vi "Select Path.vi"(8 "error in":errorcluster) -> (0 "error out":errorcluster, 1 "Save?":bool, 2 "selected path":path, 3 "Path":string)   [LabVIEW 2014, in "Data Saving.lvlib" / "Data Saver.lvclass"]
uses:
  Data Saver.lvclass
  Data Logger/PathFinder Type def.ctl
  Data Logger/Data Logger.lvclass
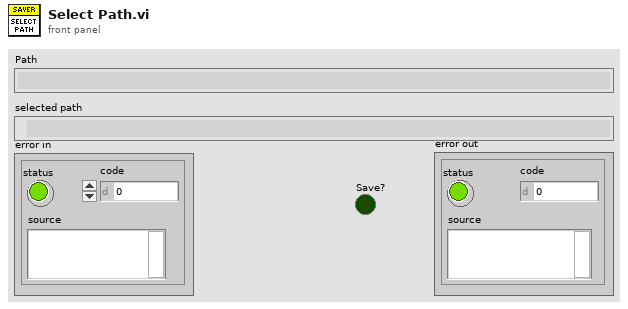
[diagram p1: front panel]
types:
  T1 = typedef "PathFinder Type def.ctl" = enum16{"Done", "Waiting"}
  T2 = cluster{"Project Number":string, "Manufacturer":string, "Model":string, "Serial":string, "Comment":string}
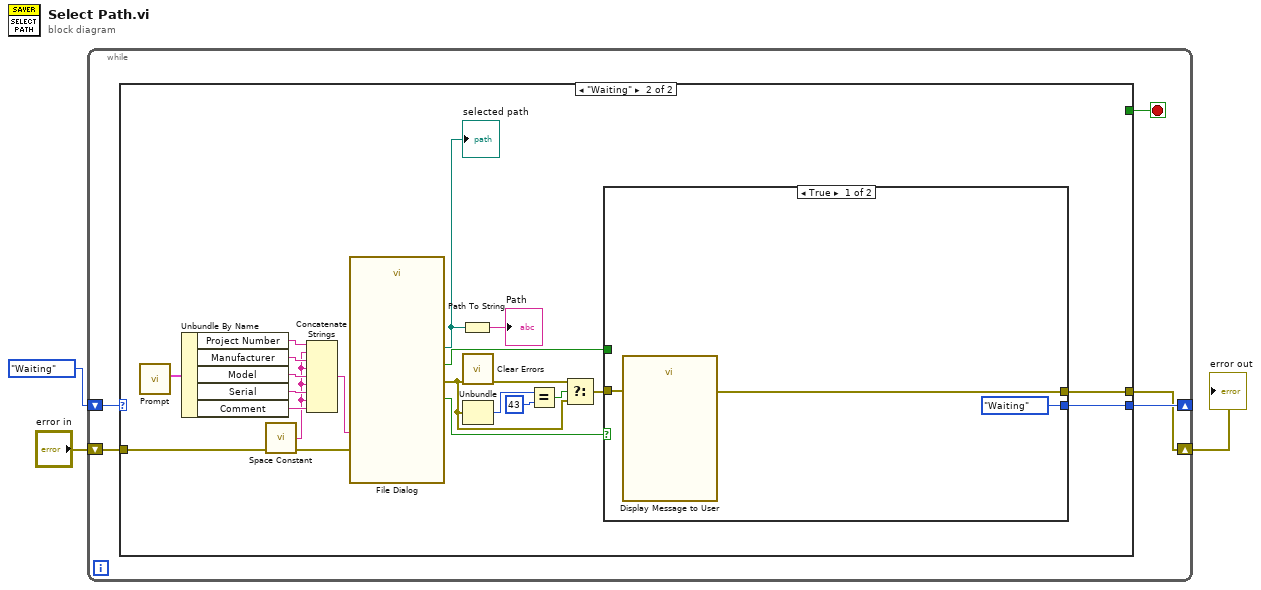
[diagram p0: block diagram]
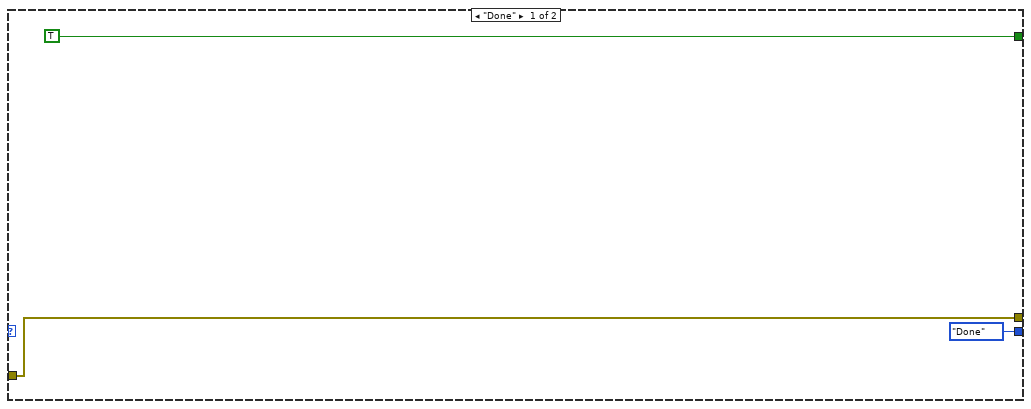
[diagram p2: hidden frame]
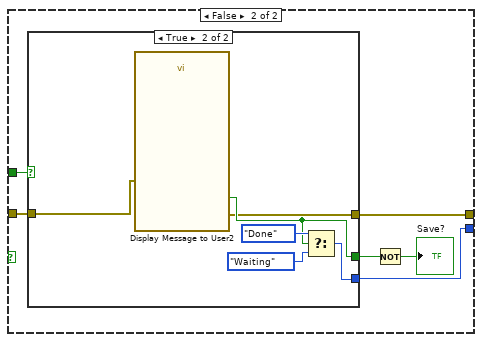
[diagram p3: hidden frame]
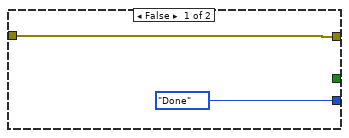
[diagram p4: hidden frame]
diagram:
  n1 = while {
    shift-right: [w6] -> _
    shift-left: PathFinder_Type_def."Waiting" -> [w8]
    shift-right: [w4] -> w1
    shift-left: "error in" -> [w5]
    stop <- w7 stop-if-true
    n2 = case shown="\"Waiting\"" w8 {
      tunnel: [TRUE _] -> w7
      tunnel: [PathFinder_Type_def."Done" w30] -> w6
      tunnel: w5 -> [w10 w19]
      tunnel: [w10 w18] -> w4
      frame "Done" {
      }
      frame "Waiting" {
        n3 = call "Prompt.vi"() -> ("Cluster"=w29:T2)  [unwired: 11 in]
        n4 = Unbundle By Name(w29) -> ("Project Number"=w28:string, "Manufacturer"=w27:string, "Model"=w26:string, "Serial"=w25:string, "Comment"=w24:string)
        n5 = call <vilib>:"Space Constant.vi"() -> ("String"=w23:string)
        n6 = Concatenate Strings(w28, w23, w27, w23, w26, w23, w25, w23, w24) -> (w22:string)
        n7 = call "File Dialog"("default name"=w22, "error in"=w19) -> ("selected path"=w21:path, "exists"=w31:bool, "cancelled"=w32:bool, "error out"=w13:errorcluster)  [unwired: 10 in]
        "selected path" <- w21
        n8 = Path To String(path=w21) -> (string=→"Path":string)
        n9 = call <vilib>:"Clear Errors.vi"("error in (no error)"=w13) -> ("error out"=w14:errorcluster)  [unwired: 5 in, 1 out]
        n10 = Unbundle(w13) -> ("code"=w17:i32)  [unwired: 2 out]
        n11 = Equal?(x=w17, y=43) -> (x = y?=w15:bool)
        n12 = Select(t=w14, s=w15, f=w13) -> (s? t:f=w12:errorcluster)
        n13 = case shown="True" w31 {
          tunnel: w32 -> [_ w41]
          tunnel: [PathFinder_Type_def."Waiting" w40] -> w30
          tunnel: w12 -> [w34 w37]
          tunnel: [w33 w36] -> w18
          frame True {
            n14 = call "Display Message to User"("error in (no error)"=w34) -> ("error out"=w33:errorcluster)  [unwired: 9 in, 1 out]
          }
          frame False {
            n15 = case shown="True" w41 {
              tunnel: [PathFinder_Type_def."Done" w47] -> w40
              tunnel: [_ w46] -> w39
              tunnel: w37 -> [w42 w45]
              tunnel: [w42 w44] -> w36
              frame False {
              }
              frame True {
                n16 = call "Display Message to User2"("error in (no error)"=w45) -> ("error out"=w44:errorcluster, "Do Not Save"=w46:bool)  [unwired: 9 in]
                n17 = Select(t=PathFinder_Type_def."Done", s=w46, f=PathFinder_Type_def."Waiting") -> (s? t:f=w47:T1)
              }
            }
            n18 = Not(x=w39) -> (.not. x?=→"Save?":bool)
          }
        }
      }
    }
  }
  "error out" <- w1
